vi "GPIB Send Receive.vi"(1 "RDY max wait, ms":u32=500, 4 "RDY when up":bool=TRUE, 5 "Data ready bit (-1 - ignore)":i32=-1, 6 "Read terminator":i16, 7 "Delay, ms":u32, 8 "error in (no error)":errorcluster, 9 "Receive count":i32=256, 10 "data string in":string, 11 "GPIB Adress":i16) -> (0 "error out":errorcluster, 2 "data string out":string, 3 "GPIB Adress out":i16)   [LabVIEW 2014]
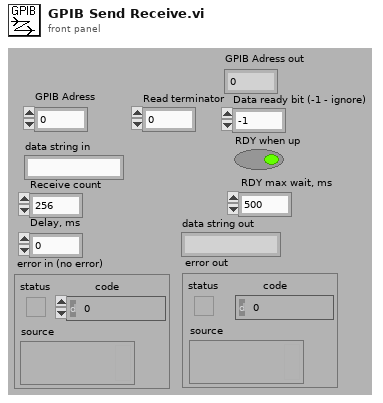
[diagram p1: front panel]
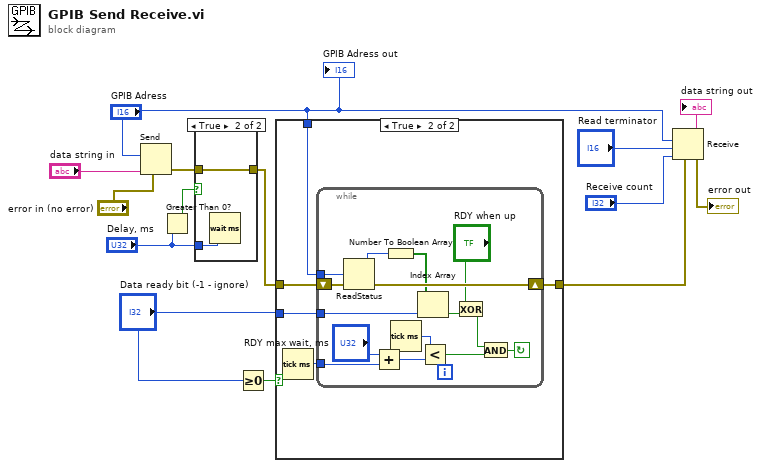
[diagram p0: block diagram]
diagram:
  n1 = Send(2:"GPIB Adress", 4:"error in (no error)", 5:"data string in") -> (8:w8:errorcluster)  [unwired: 4 out]
  n2 = Greater Than 0?(x="Delay, ms") -> (x > 0?=w9:bool)
  n3 = case shown="True" w9 {
    tunnel: w8 -> [w15 w16]
    tunnel: [w15 w16] -> w3
    tunnel: "Delay, ms" -> [_ w17]
    frame False {
    }
    frame True {
      n4 = Wait (ms)(milliseconds to wait=w17) -> ()  [unwired: 1 out]
    }
  }
  n5 = Greater Or Equal To 0?(x="Data ready bit (-1 - ignore)") -> (x >= 0?=w5:bool)
  n6 = case shown="True" w5 {
    tunnel: "GPIB Adress" -> [_ w22]
    tunnel: w3 -> [w18 w21]
    tunnel: "Data ready bit (-1 - ignore)" -> [_ w20]
    tunnel: [w18 w19] -> w1
    frame False {
    }
    frame True {
      n7 = Tick Count (ms)() -> (millisecond timer value=w23:u32)
      n8 = while {
        tunnel: w22 -> [w37]
        shift-right: [w36] -> w19
        shift-left: w21 -> [w38]
        tunnel: w23 -> [w31]
        tunnel: w20 -> [w27]
        stop <- w35 continue-if-true
        n9 = ReadStatus(3:w38, 4:w37) -> (0:w36:errorcluster, 2:w33:i16)  [unwired: 2 out]
        n10 = Add(x="RDY max wait, ms", y=w31) -> (x+y=w32:u32)
        n11 = Number To Boolean Array(number=w33) -> (Boolean array=w29:bool[])
        n12 = Tick Count (ms)() -> (millisecond timer value=w30:u32)
        n13 = Index Array(array=w29, index=w27) -> (element=w26:bool)
        n14 = Less?(x=w30, y=w32) -> (x < y?=w34:bool)
        n15 = Exclusive Or(1:w26, 2:"RDY when up") -> (0:w25:bool)
        n16 = And(x=w25, y=w34) -> (x .and. y?=w35:bool)
      }
    }
  }
  n17 = Receive(4:w1, 6:"Receive count", 7:"Read terminator", 8:"GPIB Adress") -> (0:→"error out":errorcluster, 3:→"data string out":string)  [unwired: 3 out]
  "GPIB Adress out" <- "GPIB Adress"
